vi "Constants.vi"() -> ()   [LabVIEW 2025, in "Runtime Configuration Support Example Shared.lvlib"]
doc: "Use this Global VI to access the GUIDs assigned to the page resources of the Custom Device."
uses:
  Runtime Configuration Support Example Shared.lvlib
panel:
  in  "Tab Control":enum32{"GUIDs", "Constants", "Properties"}(tab)
  in  "Inline HW":string="178d50a5-e24e-4ba6-a745-fa81ee8bee2b"
  in  "Compiled.Settings":string="Compiled.Settings"
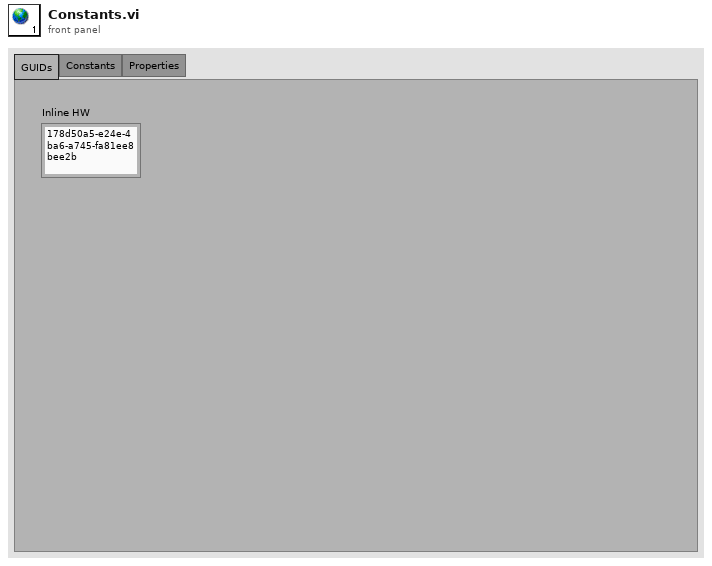
[diagram p1: front panel]
diagram:
